vi "WritePulsePositions.vi"(8 "error in (no error)":errorcluster, 10 "pulse positions array":T1[](array[typedef]), 11 "map in":T2) -> (0 "error out":errorcluster, 3 "map out":T2)   [LabVIEW 2017]
uses:
  <vilib>/addons/PointValueMap/controls/PointMap.ctl
  <vilib>/addons/InsightCM/Utilities/Analysis/Shared/controls/PulsePositions.ctl
  <vilib>/addons/PointValueMap/subVIs/Point_Write_variant.vi
  <vilib>/addons/PointValueMap/PointValueMap.lvlib
  <vilib>/addons/InsightCM/Utilities/Analysis/Shared/AnalysisHelper.lvlib
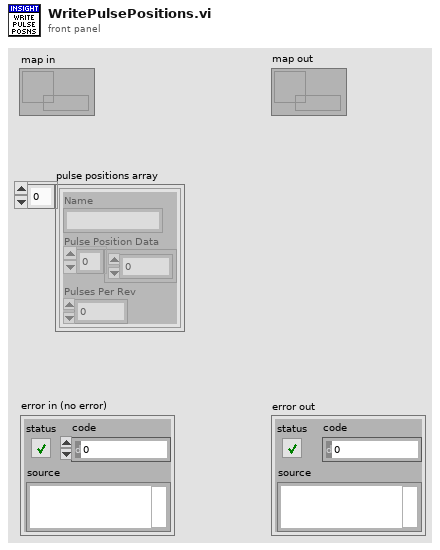
[diagram p1: front panel]
types:
  T1 = typedef "AnalysisHelper.lvlib/PulsePositions.ctl" = cluster{"Name":string, "Pulse Position Data":dbl[], "Pulses Per Rev":i32}
  T2 = typedef "PointValueMap.lvlib/PointMap.ctl" = refnum<data-value>
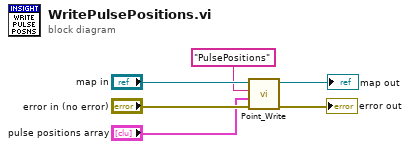
[diagram p0: block diagram]
diagram:
  n1 = call-poly <vilib>:"Point_Write.vi"("Error In"="error in (no error)", "Value"="pulse positions array", "Tag"="PulsePositions", "Map"="map in") -> ("Error Out"=→"error out":errorcluster, "Map Out"=→"map out":T2)  [unwired: 6 in]
